vi "HFRR ADV v09.vi"() -> ()   [LabVIEW 2025] (continued)
                # "password"
                # "change password logic"
                n1564 = local read "ENTER CURRENT PASSWORD"() -> (w2733:string)
                n1565 = local read "dipl pwd"() -> (w2727:string)
                n1566 = String To Byte Array(string=w2733) -> (unsigned byte array=w2735:u8[])
                n1567 = String To Byte Array(string=w2727) -> (unsigned byte array=w2728:u8[])
                n1568 = Array Size(array=w2735) -> (size(s)=w2732:i32)
                n1569 = Array Size(array=w2728) -> (size(s)=w2730:i32)
                n1570 = for {
                  N: w2732 -> [_]
                  tunnel: w2735 -> [w2759]
                  tunnel: [w2757] -> w2736 mode=indexing
                  tunnel: w2732 -> [w2751]
                  i -> [w2752]
                  n1571 = Decrement(x=w2751) -> (x-1=w2749:i32)
                  n1572 = Equal?(x=w2752, y=w2749) -> (x = y?=w2750:bool)
                  n1573 = Index Array(array=w2759, index=w2752) -> (element=w2753:u8)
                  n1574 = Number To Decimal String(number=w2753) -> (decimal integer string=w2758:string)  [unwired: 1 in]
                  n1575 = Select(t="", s=w2750, f="\r") -> (s? t:f=w2755:string)
                  n1576 = Concatenate Strings(w2758, w2755) -> (w2757:string)
                }
                n1577 = for {
                  N: w2730 -> [_]
                  tunnel: w2728 -> [w2747]
                  tunnel: [w2745] -> w2729 mode=indexing
                  tunnel: w2730 -> [w2742]
                  i -> [w2743]
                  n1578 = Decrement(x=w2742) -> (x-1=w2741:i32)
                  n1579 = Equal?(x=w2743, y=w2741) -> (x = y?=w2740:bool)
                  n1580 = Index Array(array=w2747, index=w2743) -> (element=w2746:u8)
                  n1581 = Number To Decimal String(number=w2746) -> (decimal integer string=w2744:string)  [unwired: 1 in]
                  n1582 = Select(t="", s=w2740, f="\r") -> (s? t:f=w2737:string)
                  n1583 = Concatenate Strings(w2744, w2737) -> (w2745:string)
                }
                n1584 = local read "string"() -> (w2734:string)
                n1585 = Concatenate Strings(w2729) -> (w2723:string)
                n1586 = Concatenate Strings(w2734) -> (w2731:string)
                n1587 = Concatenate Strings(w2736) -> (w2724:string)
                n1588 = Equal?(x=w2724, y=w2731) -> (x = y?=w2726:bool)
                n1589 = Equal?(x=w2724, y=w2723) -> (x = y?=w2722:bool)
                n1590 = Or(x=w2726, y=w2722) -> (x .or. y?=w2725:bool)
                n1591 = case shown="True" w2725 {
                  frame False {
                  }
                  frame True {
                    n1592 = property on="ENTER THE NEW PASSWORD" class="Str"("Visible"=TRUE) -> ()  [unwired: 2 in, 2 out]
                  }
                }
              }
            }
          }
          frame #2 {
            n1593 = String To Byte Array(string="ENTER THE NEW PASSWORD") -> (unsigned byte array=w2762:u8[])
            n1594 = Search 1D Array(1D array=w2762, element=u8 10) -> (index of element=w2766:i32)  [unwired: 1 in]
            n1595 = Index Array(array=w2762, index=w2766) -> (element=w2764:u8)
            n1596 = Equal?(x=w2764, y=10) -> (x = y?=w2761:bool)
            n1597 = case shown="False" w2761 {
              frame False {
              }
              frame True {
                n1598 = local write "EDIT"(FALSE) -> ()
                n1599 = local write "SrvM CP"(FALSE) -> ()
                n1600 = local read "ENTER THE NEW PASSWORD"() -> (w2769:string)
                n1601 = String To Byte Array(string=w2769) -> (unsigned byte array=w2774:u8[])
                n1602 = Array Size(array=w2774) -> (size(s)=w2771:i32)
                n1603 = for {
                  N: w2771 -> [_]
                  tunnel: w2774 -> [w2787]
                  tunnel: [w2784] -> w2776 mode=indexing
                  tunnel: w2771 -> [w2779]
                  i -> [w2777]
                  n1604 = Decrement(x=w2779) -> (x-1=w2780:i32)
                  n1605 = Equal?(x=w2777, y=w2780) -> (x = y?=w2781:bool)
                  n1606 = Index Array(array=w2787, index=w2777) -> (element=w2786:u8)
                  n1607 = Number To Decimal String(number=w2786) -> (decimal integer string=w2785:string)  [unwired: 1 in]
                  n1608 = Select(t="", s=w2781, f="\r") -> (s? t:f=w2778:string)
                  n1609 = Concatenate Strings(w2785, w2778) -> (w2784:string)
                }
                n1610 = local read "file path"() -> (w2768:path)
                n1611 = Concatenate Strings(w2776) -> (w2770:string)
                n1612 = Delete(path (use dialog)=w2768) -> (deleted path=w2772:path)  [unwired: 4 in, 2 out]
                n1613 = call <vilib>:"Write Characters To File.vi"("append to file? (new file:F)"=FALSE, "character string"=w2770, "file path (dialog if empty)"=w2772) -> ()  [unwired: 2 in, 1 out]
              }
            }
          }
          frame #3 {
            n1614 = case shown="True" "SrvM CP" {
              frame False {
                w2790 = ""
                n1615 = local write "ENTER CURRENT PASSWORD"(w2790) -> ()
                n1616 = local write "ENTER THE NEW PASSWORD"(w2790) -> ()
                n1617 = property on="ENTER CURRENT PASSWORD" class="Str"("Visible"=FALSE) -> ()  [unwired: 2 in, 2 out]
              }
              frame True {
                n1618 = property on="ENTER THE NEW PASSWORD" class="Str"() -> ("Visible"=w2791:bool)  [unwired: 2 in, 2 out]
                n1619 = Not(x=w2791) -> (.not. x?=w2792:bool)
                n1620 = property on="ENTER CURRENT PASSWORD" class="Str"("Visible"=w2792) -> ()  [unwired: 2 in, 2 out]
              }
            }
          }
          frame #4 {
            n1621 = String To Byte Array(string="Password") -> (unsigned byte array=w2799:u8[])
            n1622 = Search 1D Array(1D array=w2799, element=u8 10) -> (index of element=w2797:i32)  [unwired: 1 in]
            n1623 = Index Array(array=w2799, index=w2797) -> (element=w2798:u8)
            n1624 = Equal?(x=w2798, y=10) -> (x = y?=w2794:bool)
            n1625 = case shown="True" w2794 {
              frame False {
              }
              frame True {
                # "password"
                # "password"
                n1626 = local read "Password"() -> (w2812:string)
                n1627 = String To Byte Array(string=w2812) -> (unsigned byte array=w2815:u8[])
                n1628 = String To Byte Array(string="@143$\n") -> (unsigned byte array=w2801:u8[])
                n1629 = Array Size(array=w2815) -> (size(s)=w2810:i32)
                n1630 = Array Size(array=w2801) -> (size(s)=w2806:i32)
                n1631 = for {
                  N: w2810 -> [_]
                  tunnel: w2815 -> [w2849]
                  tunnel: [w2847] -> w2816 mode=indexing
                  tunnel: w2810 -> [w2844]
                  i -> [w2845]
                  n1632 = Decrement(x=w2844) -> (x-1=w2843:i32)
                  n1633 = Index Array(array=w2849, index=w2845) -> (element=w2848:u8)
                  n1634 = Equal?(x=w2845, y=w2843) -> (x = y?=w2842:bool)
                  n1635 = Number To Decimal String(number=w2848) -> (decimal integer string=w2846:string)  [unwired: 1 in]
                  n1636 = Select(t="", s=w2842, f="\r") -> (s? t:f=w2839:string)
                  n1637 = Concatenate Strings(w2846, w2839) -> (w2847:string)
                }
                n1638 = for {
                  N: w2806 -> [_]
                  tunnel: w2801 -> [w2860]
                  tunnel: [w2858] -> w2804 mode=indexing
                  tunnel: w2806 -> [w2855]
                  i -> [w2856]
                  n1639 = Decrement(x=w2855) -> (x-1=w2854:i32)
                  n1640 = Index Array(array=w2860, index=w2856) -> (element=w2859:u8)
                  n1641 = Equal?(x=w2856, y=w2854) -> (x = y?=w2853:bool)
                  n1642 = Number To Decimal String(number=w2859) -> (decimal integer string=w2857:string)  [unwired: 1 in]
                  n1643 = Select(t="", s=w2853, f="\r") -> (s? t:f=w2850:string)
                  n1644 = Concatenate Strings(w2857, w2850) -> (w2858:string)
                }
                n1645 = local read "file path"() -> (w2800:path)
                n1646 = call <vilib>:"Read Characters From File.vi"("file path (dialog if empty)"=w2800) -> ("character string"=w2814:string)  [unwired: 5 in, 3 out]
                "string" <- w2814
                n1647 = flat-sequence {
                  tunnel: [w2817] -> w2811
                  frame #0 {
                    w2817 = ""
                    n1648 = local write "Password"(w2817) -> ()
                  }
                }
                n1649 = Concatenate Strings(w2804) -> (w2805:string)
                n1650 = Concatenate Strings(w2814) -> (w2813:string)
                n1651 = Concatenate Strings(w2816) -> (w2808:string)
                n1652 = Equal?(x=w2808, y=w2813) -> (x = y?=w2803:bool)
                n1653 = Equal?(x=w2808, y=w2805) -> (x = y?=w2809:bool)
                n1654 = Or(x=w2803, y=w2809) -> (x .or. y?=w2802:bool)
                "x = y?" <- w2802
                n1655 = case shown="True" w2802 {
                  selector: w2802 -> [w2819 _]
                  tunnel: w2811 -> [_ _]
                  frame False {
                    n1656 = And(x=w2819, y=TRUE ("Visible")) -> (x .and. y?=w2820:bool)
                    n1657 = property on="message" class="Str"("Visible"=w2820) -> ()  [unwired: 2 in, 2 out]
                  }
                  frame True {
                    n1658 = control-ref of="This VI"() -> (w2831:refnum<vi>)
                    n1659 = property class="VI"(reference=w2831) -> (reference out=w2822:refnum<vi>, error out=w2826:errorcluster, "Panel"=w2830:refnum<vi>)  [unwired: 1 in]
                    n1660 = property on="message" class="Str"("Visible"=FALSE) -> ()  [unwired: 2 in, 2 out]
                    n1661 = property class="Pnl"(reference=w2830, error in=w2826) -> (reference out=w2824:refnum<vi>, error out=w2827:errorcluster, "Panes[]"=w2829:refnum<vi>[])
                    n1662 = for {
                      tunnel: w2829 -> [w2838] mode=indexing
                      tunnel: T17."Always On" ("Horizontal Scrollbar Visibility") -> [w2837]
                      tunnel: w2827 -> [w2834]
                      tunnel: [w2833] -> w2825
                      n1663 = property class="Pane"(reference=w2838, error in=w2834, "HorizScrollbarVisibility"=w2837) -> (reference out=w2835:refnum<vi>, error out=w2836:errorcluster)
                      n1664 = Close Reference(reference=w2835, error in (no error)=w2836) -> (error out=w2833:errorcluster)
                    }
                    n1665 = Close Reference(reference=w2824, error in (no error)=w2825) -> (error out=w2823:errorcluster)
                    n1666 = Close Reference(reference=w2822, error in (no error)=w2823) -> (error out=→"error out 6":errorcluster)
                  }
                }
              }
            }
          }
        }
        n1667 = local read "x = y?"() -> (w2659:bool)
        n1668 = local read "HUMIDITY: 2"() -> (w2661:dbl)
        n1669 = local read "HUMIDITY:"() -> (w2660:dbl)
        n1670 = property on="Port 2 Error" class="Clust (strict)"("Visible"="EDIT") -> ()  [unwired: 2 in, 2 out]
        n1671 = property on="Port 1 Error" class="Clust (strict)"("Visible"="EDIT") -> ()  [unwired: 2 in, 2 out]
        n1672 = case shown="True" "SrvM CP 2" {
          frame False {
          }
          frame True {
            n1673 = local write "SrvM CP 2"(FALSE ("SrvM CP 2")) -> ()
            n1674 = local read "HUMIDITY: 2"() -> (w2700:dbl)
            n1675 = local read "TEMP INTERCEPT: 2"() -> (w2699:dbl)
            n1676 = local read "DISPLACEMENT : 4"() -> (w2703:dbl)
            n1677 = local read "TEMPERATURE : 2"() -> (w2702:dbl)
            n1678 = local read "STROKE GAIN : 2"() -> (w2704:dbl)
            n1679 = local read "FRIC. FORCE : 2"() -> (w2705:dbl)
            n1680 = local read "AIR TEMP INTERCEPT: 2"() -> (w2698:dbl)
            n1681 = local read "AIR TEMPERATURE : 2"() -> (w2701:dbl)
            n1682 = local write "HUMIDITY:"(w2700) -> ()
            n1683 = local write "AIR TEMP INTERCEPT:"(w2699) -> ()
            n1684 = local write "TEMPERATURE :"(w2702) -> ()
            n1685 = local write "FRIC. FORCE :"(w2705) -> ()
            n1686 = local write "STROKE GAIN :"(w2704) -> ()
            n1687 = local write "DISPLACEMENT :"(w2703) -> ()
            n1688 = local write "AIR TEMPERATURE :"(w2701) -> ()
            n1689 = local write "TEMP INTERCEPT:"(w2698) -> ()
          }
        }
        n1690 = case shown="True" "SAVE" {
          frame False {
          }
          frame True {
            n1691 = stacked-sequence {
              seq-local: [w2877 _ _] -> [_ w3041 _]
              frame #0 {
                (unwired) i16 5 ("precision (6)")
                # "[CH1]    - FF\n[CH2]   - TEMPERATURE\n[CH3]    - Humidity\n[CH4]    - AIR TEMP\n[CH5]\\- Visa Uno\n[CH6] \\- Visa Due\n[CH7]  \\- file path\n[CH8]   - Displacement Gain\n[CHA]   - Stroke Gain\n[CHB]   - Stroke PID Gain\n[CHC]   -Language Selection\n[CHD]   -Power +\n[CHE]   -Power_\n[CHF]   -Heater\n[CHG]   -Humidity Wet\n[CHH]   -Humidity Dry\n[CHI]   -Integral Time"
                n1692 = local read "Stroke PID Gains"() -> (w2928:T8)
                n1693 = Unbundle By Name(w2928) -> ("Proportional Gain (Kc)"=w2927:dbl, "Integral Time (Ti, min)"=w2869:dbl)
                n1694 = Number To Fractional String(number=w2869, width (-)=i16 10 ("precision (6)"), precision (6)=i16 5) -> (F-format string=w2873:string)  [unwired: 1 in]
                n1695 = local read "Language Selection"() -> (w2925:enum16{"English", "Russian"})
                n1696 = local read "CH-HUMIDITY WET"() -> (w2883:u16)
                n1697 = local read "CH-HUMIDITY DRY"() -> (w2880:u16)
                n1698 = local read "STROKE GAIN :"() -> (w2861:dbl)
                n1699 = local read "CH-POWER +"() -> (w2892:u16)
                n1700 = local read "CH-POWER -"() -> (w2889:u16)
                n1701 = local read "CH-HEATER"() -> (w2886:u16)
                n1702 = local read "AIR TEMPERATURE :"() -> (w2864:dbl)
                n1703 = Concatenate Strings("[CHI]" ("string"), w2873, "-Integral Time " ("string"), "\r") -> (w2870:string)
                n1704 = local read "DISPLACEMENT :"() -> (w2862:dbl)
                n1705 = local read "TEMPERATURE :"() -> (w2865:dbl)
                n1706 = local read "FRIC. FORCE :"() -> (w2866:dbl)
                n1707 = local read "HUMIDITY:"() -> (w2863:dbl)
                n1708 = Path To String(path="File Path") -> (string=w2950:string)
                n1709 = Number To Fractional String(number=w2861, width (-)=i16 10 ("precision (6)"), precision (6)=i16 5) -> (F-format string=w2941:string)  [unwired: 1 in]
                n1710 = Number To Fractional String(number=w2927, width (-)=i16 10 ("precision (6)"), precision (6)=i16 5) -> (F-format string=w2929:string)  [unwired: 1 in]
                n1711 = Number To Fractional String(number=w2925, width (-)=i16 10 ("precision (6)"), precision (6)=i16 5) -> (F-format string=w2921:string)  [unwired: 1 in]
                n1712 = Number To Fractional String(number=w2892, width (-)=i16 10 ("precision (6)"), precision (6)=i16 5) -> (F-format string=w2915:string)  [unwired: 1 in]
                n1713 = Number To Fractional String(number=w2889, width (-)=i16 10 ("precision (6)"), precision (6)=i16 5) -> (F-format string=w2912:string)  [unwired: 1 in]
                n1714 = Number To Fractional String(number=w2886, width (-)=i16 10 ("precision (6)"), precision (6)=i16 5) -> (F-format string=w2907:string)  [unwired: 1 in]
                n1715 = Number To Fractional String(number=w2883, width (-)=i16 10 ("precision (6)"), precision (6)=i16 5) -> (F-format string=w2904:string)  [unwired: 1 in]
                n1716 = Number To Fractional String(number=w2880, width (-)=i16 10 ("precision (6)"), precision (6)=i16 5) -> (F-format string=w2899:string)  [unwired: 1 in]
                n1717 = local read "Com Port 1"() -> (w2868:refnum<visa-resource-name>)
                n1718 = local read "Com Port 2"() -> (w2867:refnum<visa-resource-name>)
                n1719 = Concatenate Strings(w2950, "\\" ("string")) -> (w2949:string)
                n1720 = Number To Fractional String(number=w2866, width (-)=i16 10 ("precision (6)"), precision (6)=i16 5) -> (F-format string=w2982:string)  [unwired: 1 in]
                n1721 = Number To Fractional String(number=w2865, width (-)=i16 10 ("precision (6)"), precision (6)=i16 5) -> (F-format string=w2981:string)  [unwired: 1 in]
                n1722 = Number To Fractional String(number=w2863, width (-)=i16 10 ("precision (6)"), precision (6)=i16 5) -> (F-format string=w2975:string)  [unwired: 1 in]
                n1723 = Number To Fractional String(number=w2864, width (-)=i16 10 ("precision (6)"), precision (6)=i16 5) -> (F-format string=w2969:string)  [unwired: 1 in]
                n1724 = Number To Fractional String(number=w2862, width (-)=i16 10 ("precision (6)"), precision (6)=i16 5) -> (F-format string=w2942:string)  [unwired: 1 in]
                n1725 = Concatenate Strings("[CHA]" ("string"), w2941, "- Stroke Gain" ("string"), "\r") -> (w2935:string)
                n1726 = Concatenate Strings("[CHB]" ("string"), w2929, "- Stroke PID Gain" ("string"), "\r") -> (w2926:string)
                n1727 = Concatenate Strings("[CHC]" ("string"), w2921, "-Language Selection" ("string"), "\r") -> (w2918:string)
                n1728 = Concatenate Strings("[CHD]" ("string"), w2915, "-Power +" ("string"), "\r") -> (w2897:string)
                n1729 = Concatenate Strings("[CHG]" ("string"), w2904, "-Humidity Wet" ("string"), "\r") -> (w2894:string)
                n1730 = Concatenate Strings("[CHH]" ("string"), w2899, "-Humidity Dry" ("string"), "\r") -> (w2893:string)
                n1731 = Concatenate Strings("[CH1]" ("string"), w2982, " - FF" ("string"), "\r") -> (w2980:string)
                n1732 = Concatenate Strings("[CH2]" ("string"), w2981, " - TEMPERATURE" ("string"), "\r") -> (w2979:string)
                n1733 = Concatenate Strings("[CH3]" ("string"), w2975, " - Humidity" ("string"), "\r") -> (w2972:string)
                n1734 = Concatenate Strings("[CH4]" ("string"), w2969, " - AIR TEMP" ("string"), "\r") -> (w2965:string)
                n1735 = Concatenate Strings("[CH5]" ("string"), w2868, "- Visa Uno" ("string"), "\r") -> (w2958:string)
                n1736 = Concatenate Strings("[CH6]" ("string"), w2867, "- Visa Due" ("string"), "\r") -> (w2953:string)
                n1737 = Concatenate Strings("[CH7]" ("string"), w2949, "- file path" ("string"), "\r") -> (w2952:string)
                n1738 = Concatenate Strings("[CH8]" ("string"), w2942, "- Displacement Gain" ("string"), "\r") -> (w2945:string)
                n1739 = Concatenate Strings("[CHE]" ("string"), w2912, "-Power_" ("string"), "\r") -> (w2896:string)
                n1740 = Concatenate Strings("[CHF]" ("string"), w2907, "-Heater" ("string"), "\r") -> (w2895:string)
                n1741 = Concatenate Strings(w2980, w2979, w2972, w2965, w2958, w2953, w2952, w2945, w2935, w2926, w2918, w2897, w2896, w2895, w2894, w2893, w2870) -> (w2877:string)
                "gain" <- w2877
              }
              frame #1 {
                n1742 = local read "Camera Port :"() -> (w2994:string)
                n1743 = local read "TEMP INTERCEPT:"() -> (w3003:dbl)
                n1744 = local read "Humidity :"() -> (w3002:refnum<visa-resource-name>)
                n1745 = local read "AIR TEMP INTERCEPT:"() -> (w3004:dbl)
                n1746 = local read "LvdtOff"() -> (w3006:dbl)
                n1747 = Number To Fractional String(number=w3003, width (-)=i16 10 ("precision (6)"), precision (6)=i16 5) -> (F-format string=w3029:string)  [unwired: 1 in]
                n1748 = local read "Com Port 3"() -> (w3013:refnum<visa-resource-name>)
                n1749 = Concatenate Strings("[CH8]" ("string"), w2994, "- Visa Camera" ("string"), "\r") -> (w2993:string)
                n1750 = Concatenate Strings("[CH7]" ("string"), w3002, "- Visa Humidity" ("string"), "\r") -> (w2998:string)
                n1751 = Number To Fractional String(number=w3004, width (-)=i16 10 ("precision (6)"), precision (6)=i16 5) -> (F-format string=w3036:string)  [unwired: 1 in]
                n1752 = Number To Fractional String(number=w3006, width (-)=i16 10 ("precision (6)"), precision (6)=i16 5) -> (F-format string=w3010:string)  [unwired: 1 in]
                n1753 = Concatenate Strings("[CHK]" ("string"), w3029, "-TEMP INTERCEPT" ("string"), "\r") -> (w3025:string)
                n1754 = Concatenate Strings("[SNO]" ("string"), "S.NO", "-" ("string"), "\r") -> (w3021:string)
                n1755 = Concatenate Strings("[CHI]" ("string"), w3010, "-LVDT Position Offset" ("string"), "\r") -> (w3005:string)
                n1756 = Concatenate Strings("[CHJ]" ("string"), w3036, "-AIR TEMP INTERCEPT" ("string"), "\r") -> (w3026:string)
                n1757 = Concatenate Strings("[CHL]" ("string"), w3013, "- Visa humid" ("string"), "\r") -> (w3016:string)
                n1758 = String To Path(string="C:\\LAB-IQ\\calibrate WO 2465.dcf") -> (path=w3014:path)
                n1759 = Concatenate Strings(w3041, w3026, w3025, w3021, w3016, w3005, w2998, w2993) -> (w3040:string)
                n1760 = call <vilib>:"Write Characters To File.vi"("append to file? (new file:F)"=FALSE, "character string"=w3040, "file path (dialog if empty)"=w3014) -> ()  [unwired: 2 in, 1 out]
              }
              frame #2 {
                n1761 = local write "Lan flag"(0.0 ("Lan flag")) -> ()
                n1762 = local write "conststatus"(0.0 ("rpm value : 2")) -> ()
                n1763 = local write "SAVE"(FALSE ("OK Button 14")) -> ()
                n1764 = local write "Re-Initialise"(TRUE ("Re-Initialise")) -> ()
              }
            }
          }
        }
        n1765 = And(x="EDIT", y=w2659) -> (x .and. y?=w2657:bool)
        n1766 = local read "DISPLACEMENT : 4"() -> (w2670:dbl)
        n1767 = local read "TEMPERATURE : 2"() -> (w2668:dbl)
        n1768 = local read "STROKE GAIN : 2"() -> (w2674:dbl)
        n1769 = local read "DISPLACEMENT :"() -> (w2669:dbl)
        n1770 = local read "FRIC. FORCE : 2"() -> (w2677:dbl)
        n1771 = local read "TEMPERATURE :"() -> (w2666:dbl)
        n1772 = local read "STROKE GAIN :"() -> (w2673:dbl)
        n1773 = local read "FRIC. FORCE :"() -> (w2676:dbl)
        n1774 = case shown="True" w2657 {
          tunnel: [u8 2 ("Disabled") u8 0 ("Disabled")] -> w2656
          tunnel: [w3046 TRUE ("Visible")] -> w2655
          frame False {
            w3046 = FALSE ("Visible")
            n1775 = local write "EDIT 2"(w3046) -> ()
          }
          frame True {
          }
        }
        n1776 = Subtract(x=w2661, y=w2660) -> (x-y=w2662:dbl)
        n1777 = local read "AIR TEMPERATURE : 2"() -> (w2665:dbl)
        n1778 = local read "AIR TEMPERATURE :"() -> (w2664:dbl)
        n1779 = Divide(x=w2662, y=w2660) -> (x/y=w2684:dbl)
        n1780 = Subtract(x=w2677, y=w2676) -> (x-y=w2675:dbl)
        n1781 = Subtract(x=w2668, y=w2666) -> (x-y=w2667:dbl)
        n1782 = Subtract(x=w2674, y=w2673) -> (x-y=w2672:dbl)
        n1783 = Subtract(x=w2670, y=w2669) -> (x-y=w2671:dbl)
        n1784 = Subtract(x=w2665, y=w2664) -> (x-y=w2663:dbl)
        n1785 = Divide(x=w2675, y=w2676) -> (x/y=w2695:dbl)
        n1786 = Divide(x=w2667, y=w2666) -> (x/y=w2688:dbl)
        n1787 = Divide(x=w2672, y=w2673) -> (x/y=w2692:dbl)
        n1788 = Divide(x=w2671, y=w2669) -> (x/y=w2691:dbl)
        n1789 = Multiply(x=w2684, y=100.0) -> (x*y=→"HUMIDITY  Calibration Error":dbl)
        n1790 = Divide(x=w2663, y=w2664) -> (x/y=w2687:dbl)
        n1791 = Multiply(x=w2695, y=100.0) -> (x*y=→"FRIC. FORCE Calibration Error":dbl)
        n1792 = Multiply(x=w2688, y=100.0) -> (x*y=→"TEMPERATURE  Calibration Error":dbl)
        n1793 = Multiply(x=w2692, y=100.0) -> (x*y=→"STROKE Calibration Error":dbl)
        n1794 = Multiply(x=w2691, y=100.0) -> (x*y=→"DISPLACEMENT  Calibration Error":dbl)
        n1795 = property on="EDIT 2" class="Bool (strict)"("Visible"=w2655) -> ()  [unwired: 2 in, 2 out]
        n1796 = property on="SAVE" class="Bool (strict)"("Visible"=w2655) -> ()  [unwired: 2 in, 2 out]
        n1797 = property on="SrvM CP" class="Bool (strict)"("Disabled"=w2656) -> ()  [unwired: 2 in, 2 out]
        n1798 = property on="visa due" class="CmbBox"("Disabled"=w2656) -> ()  [unwired: 2 in, 2 out]
        n1799 = property on="LvdtOff" class="DigNum (strict)"("Disabled"=w2656) -> ()  [unwired: 2 in, 2 out]
        n1800 = property on="File Path" class="Path"("Disabled"=w2656) -> ()  [unwired: 2 in, 2 out]
        n1801 = Multiply(x=w2687, y=100.0) -> (x*y=→"AIR TEMPERATURE  Calibration Error":dbl)
        n1802 = property on="Tab Control" class="TabCtl (strict)"("Visible"=w2655) -> ()  [unwired: 2 in, 2 out]
        n1803 = property on="Language Selection" class="Enum (strict)"("Visible"=w2655) -> ()  [unwired: 2 in, 2 out]
        n1804 = property on="Tab Control 7" class="TabCtl (strict)"("Disabled"=w2656) -> ()  [unwired: 2 in, 2 out]
        n1805 = property on="AIR TEMP INTERCEPT:" class="DigNum (strict)"("Disabled"=w2656) -> ()  [unwired: 2 in, 2 out]
        n1806 = property on="CH-POWER -" class="DigNum (strict)"("Disabled"=w2656) -> ()  [unwired: 2 in, 2 out]
        n1807 = property on="CH-POWER +" class="DigNum (strict)"("Disabled"=w2656) -> ()  [unwired: 2 in, 2 out]
        n1808 = property on="AIR TEMPERATURE :" class="DigNum (strict)"("Disabled"=w2656) -> ()  [unwired: 2 in, 2 out]
        n1809 = property on="STROKE GAIN :" class="DigNum (strict)"("Disabled"=w2656) -> ()  [unwired: 2 in, 2 out]
        n1810 = property on="SPEED OUT:" class="DigNum (strict)"("Disabled"=w2656) -> ()  [unwired: 2 in, 2 out]
        n1811 = property on="CH-HUMIDITY DRY" class="DigNum (strict)"("Disabled"=w2656) -> ()  [unwired: 2 in, 2 out]
        n1812 = property on="HUMIDITY:" class="DigNum (strict)"("Disabled"=w2656) -> ()  [unwired: 2 in, 2 out]
        n1813 = property on="CH-HUMIDITY WET" class="DigNum (strict)"("Disabled"=w2656) -> ()  [unwired: 2 in, 2 out]
        n1814 = property on="Stroke PID Gains" class="Clust (strict)"("Disabled"=w2656) -> ()  [unwired: 2 in, 2 out]
        n1815 = property on="TEMPERATURE :" class="DigNum (strict)"("Disabled"=w2656) -> ()  [unwired: 2 in, 2 out]
        n1816 = property on="DISPLACEMENT :" class="DigNum (strict)"("Disabled"=w2656) -> ()  [unwired: 2 in, 2 out]
        n1817 = property on="CH-HEATER" class="DigNum (strict)"("Disabled"=w2656) -> ()  [unwired: 2 in, 2 out]
        n1818 = property on="TEMP INTERCEPT:" class="DigNum (strict)"("Disabled"=w2656) -> ()  [unwired: 2 in, 2 out]
        n1819 = property on="FRIC. FORCE :" class="DigNum (strict)"("Disabled"=w2656) -> ()  [unwired: 2 in, 2 out]
      }
    }
    n1820 = local read "RUN"() -> (w2051:bool)
    n1821 = local read "RUN"() -> (w2049:bool)
    n1822 = disable-structure shown="Disabled" {
      disable-tunnel: [w2066 _] -> w2031
      disable-tunnel: [w2065 _] -> w2029
      frame Disabled {
        n1823 = local read "Temperature before test"() -> (w2059:dbl)
        n1824 = local read "Temperature after test"() -> (w2072:dbl)
        n1825 = case shown="True" "Save Results" {
          frame False {
          }
          frame True {
            w2088 = "\r"
            n1826 = local write "Save Results"(FALSE ("OK Button 5")) -> ()
            n1827 = local read "Temperature before test"() -> (w2126:dbl)
            n1828 = local read "Temperature after test"() -> (w2128:dbl)
            n1829 = local read "Humidity before test"() -> (w2125:dbl)
            n1830 = local read "Humidity after test"() -> (w2127:dbl)
            n1831 = local read "WS1.4"() -> (w2132:dbl)
            n1832 = local read "AVP"() -> (w2130:dbl)
            n1833 = Number To Fractional String(number=w2132, width (-)=i16 6, precision (6)=i16 1) -> (F-format string=w2092:string)  [unwired: 1 in]
            n1834 = local read "MWSD"() -> (w2129:dbl)
            n1835 = local read "String"() -> (w2121:string)
            n1836 = local read "FILE"() -> (w2124:string)
            n1837 = local read "HCF"() -> (w2131:dbl)
            n1838 = Number To Fractional String(number=w2125, width (-)=i16 6, precision (6)=i16 1) -> (F-format string=w2117:string)  [unwired: 1 in]
            n1839 = Number To Fractional String(number=w2126, width (-)=i16 6, precision (6)=i16 1) -> (F-format string=w2114:string)  [unwired: 1 in]
            n1840 = Number To Fractional String(number=w2127, width (-)=i16 6, precision (6)=i16 1) -> (F-format string=w2110:string)  [unwired: 1 in]
            n1841 = Number To Fractional String(number=w2128, width (-)=i16 6, precision (6)=i16 1) -> (F-format string=w2106:string)  [unwired: 1 in]
            n1842 = Number To Fractional String(number=w2130, width (-)=i16 6, precision (6)=i16 3) -> (F-format string=w2099:string)  [unwired: 1 in]
            n1843 = Concatenate Strings(w2121, w2124) -> (w2143:string)
            n1844 = Number To Fractional String(number=w2129, width (-)=i16 6, precision (6)=i16 1) -> (F-format string=w2103:string)  [unwired: 1 in]
            n1845 = Number To Fractional String(number=w2131, width (-)=i16 6, precision (6)=i16 2) -> (F-format string=w2097:string)  [unwired: 1 in]
            n1846 = Concatenate Strings("(" ("string"), w2092, ")Microns" ("string")) -> (w2091:string)
            n1847 = local read "REMARKS"() -> (w2123:string)
            "REMARKS 2" <- w2123
            n1848 = Concatenate Strings("(" ("string"), w2117, " ) % RH," ("string")) -> (w2118:string)
            n1849 = Concatenate Strings(w2097, ")" ("string")) -> (w2095:string)
            n1850 = Concatenate Strings("(" ("string"), w2114, ")  Deg C ," ("string")) -> (w2113:string)
            n1851 = Concatenate Strings("(" ("string"), w2110, " ) % RH," ("string")) -> (w2109:string)
            n1852 = Concatenate Strings("(" ("string"), w2106, ")  Deg C ," ("string")) -> (w2105:string)
            n1853 = Concatenate Strings("(" ("string"), w2103, ")  Microns," ("string")) -> (w2102:string)
            n1854 = Concatenate Strings("(" ("string"), w2099, ")  kPa," ("string")) -> (w2089:string)
            n1855 = Concatenate Strings(w2143, ".dwm" ("Substring")) -> (w2141:string)
            n1856 = String To Path(string=w2141) -> (path=w2140:path)
            n1857 = Concatenate Strings(w2123, w2088, " Humidity before test= " ("Substring"), w2118, w2088, " Temperature before test = " ("Substring"), w2113, w2088, " Humidity after test= " ("Substring"), w2109, w2088, "Temperature after test = " ("Substring"), w2105, w2088, "MSD = " ("Substring"), w2102, w2088, "  AVP = " ("Substring"), w2089, w2088, "  HCF                     =( " ("Substring"), w2095, w2088, " WS1.4                  = " ("Substring"), w2091, w2088) -> (w2087:string)
            "data" <- w2087
            n1858 = call <vilib>:"Write Characters To File.vi"("append to file? (new file:F)"=FALSE, "character string"=w2087, "file path (dialog if empty)"=w2140) -> ()  [unwired: 2 in, 1 out]
            n1859 = Match Pattern(string=w2087, regular expression="!") -> (after substring=→"export":string)  [unwired: 1 in, 3 out]
          }
        }
        n1860 = Add(x=231.864, y=w2059) -> (x+y=w2056:dbl)
        n1861 = Add(x=231.864, y=w2072) -> (x+y=w2069:dbl)
        n1862 = Divide(x=1705.984, y=w2056) -> (x/y=w2057:dbl)
        n1863 = Divide(x=1705.984, y=w2069) -> (x/y=w2070:dbl)
        n1864 = local read "Humidity before test"() -> (w2061:dbl)
        n1865 = local read "Humidity after test"() -> (w2074:dbl)
        n1866 = Subtract(x=8.017352 ("y"), y=w2057) -> (x-y=w2083:dbl)
        n1867 = Subtract(x=8.017352 ("y"), y=w2070) -> (x-y=w2077:dbl)
        n1868 = expression code="10**y"(w2083) -> (w2063:dbl)
        n1869 = expression code="10**y"(w2077) -> (w2076:dbl)
        n1870 = Multiply(x=w2061, y=w2063) -> (x*y=w2062:dbl)
        n1871 = Multiply(x=w2074, y=w2076) -> (x*y=w2075:dbl)
        n1872 = Divide(x=w2062, y=750.0) -> (x/y=w2078:dbl)
        n1873 = Divide(x=w2075, y=750.0) -> (x/y=w2079:dbl)
        n1874 = Add(x=w2078, y=w2079) -> (x+y=w2080:dbl)
        n1875 = Divide(x=w2080, y=2.0) -> (x/y=w2082:dbl)
        n1876 = local write "AVP"(w2082) -> ()
        n1877 = Subtract(x=1.4, y=w2082) -> (x-y=w2065:dbl)
        n1878 = local read "HCF"() -> (w2066:dbl)
      }
      frame Enabled {
      }
    }
    n1879 = case shown="True" "EDIT 3" {
      frame False {
      }
      frame True {
        n1880 = local write "EDIT 3"(FALSE ("EDIT 3")) -> ()
        n1881 = local write "Main Tab"(T2."About" ("Main Tab")) -> ()
      }
    }
    n1882 = case shown="True" w2037 {
      frame False {
      }
      frame True {
        n1883 = local write "Re-Initialise"(FALSE ("Re-Initialise")) -> ()
      }
    }
    n1884 = case shown="False" w2051 {
      frame False {
        n1885 = local read "stopT"() -> (w3053:bool)
        n1886 = case shown="True" w3053 {
          frame False {
          }
          frame True {
            w3054 = FALSE
            n1887 = local write "stopT"(w3054) -> ()
            n1888 = local write "st enable"(w3054) -> ()
          }
        }
      }
      frame True {
        "stopT" <- TRUE
      }
    }
    n1889 = case shown="True" w2049 {
      frame False {
      }
      frame True {
      }
    }
    n1890 = case shown="True" w2039 {
      frame False {
        n1891 = property on="Password 2" class="Str"("Visible"=FALSE) -> ()  [unwired: 2 in, 2 out]
        n1892 = local write "Password 2"("" ("Password")) -> ()
      }
      frame True {
        n1893 = property on="Password 2" class="Str"("Visible"=TRUE) -> ()  [unwired: 2 in, 2 out]
        n1894 = Equal?(x="Password 2", y="HFRR1234") -> (x = y?=w2172:bool)
        n1895 = case shown="True" w2172 {
          tunnel: "Password 2" -> [w2175 _]
          frame False {
            n1896 = String Length(string=w2175) -> (length=w2176:i32)
            n1897 = Greater Than 0?(x=w2176) -> (x > 0?=w2174:bool)
            n1898 = case shown="False" w2174 {
              frame False {
                n1899 = property on="Password 2" class="Str"("Caption.Text"="Password (Advance Setting)") -> ()  [unwired: 2 in, 2 out]
              }
              frame True {
                n1900 = property on="Password 2" class="Str"("Caption.Text"="Incorrect Password!") -> ()  [unwired: 2 in, 2 out]
              }
            }
          }
          frame True {
            n1901 = local write "EDIT 2"(FALSE ("EDIT 2")) -> ()
            n1902 = local write "Password 2"("" ("Password")) -> ()
            n1903 = local write "Main Tab"(T2."Advance" ("Main Tab")) -> ()
            n1904 = local write "Main Dashboard Buttons"(T1."Advance" ("Main Dashboard Buttons")) -> ()
          }
        }
      }
    }
    n1905 = case shown="True" "Prog Uno" {
      frame False {
      }
      frame True {
        n1906 = stacked-sequence {
          frame #0 {
            n1907 = Delete(path (use dialog)=path "C:/LAB-IQ-NXT/UNOCOMPILE.bat" ("working directory")) -> ()  [unwired: 4 in, 3 out]
          }
          frame #1 {
            n1908 = local read "Com Port 1"() -> (w2637:refnum<visa-resource-name>)
            n1909 = Concatenate Strings("cmd.exe /c \"mode " ("command line"), w2637, ":1200,n,8,1\"\n" ("command line")) -> (w2642:string)
            n1910 = Concatenate Strings(w2642, "CD\\\nCD WinDucom\navrdude -C avrdude.conf -v -patmega328p -carduino -P" ("command line"), w2637, " -b115200 -D -Uflash:w:UNO_V20.hex:i\n" ("command line"), "\r") -> (w2644:string)
            "STR" <- w2644
            n1911 = call <vilib>:"Write Characters To File.vi"("append to file? (new file:F)"=FALSE, "character string"=w2644, "file path (dialog if empty)"=path "C:/LAB-IQ/UNOCOMPILE.bat" ("working directory")) -> ()  [unwired: 2 in, 1 out]
          }
          frame #2 {
            n1912 = disable-structure shown="Disabled" {
              frame Disabled {
                w2648 = "cmd.exe  /c \"C:\\LAB-IQ-NXT\\UNOCOMPILE.bat\"" ("string")
                n1913 = local write "Prog Uno"(FALSE ("run minimized? (F)")) -> ()
                n1914 = call <vilib>:"System Exec.vi"("expected output size  (4096)"=u32 65535, "run minimized? (F)"=FALSE, "wait until completion? (T)"=TRUE ("run minimized? (F)"), "working directory"=path "C:/LAB-IQ-NXT", "standard input"=w2648, "command line"=w2648) -> ("error out"=w2647:errorcluster, "standard output"=→"String 42":string)  [unwired: 2 in, 2 out]
                "error out 3" <- w2647
                n1915 = flat-sequence {
                  tunnel: w2647 -> [_]
                  frame #0 {
                  }
                }
              }
              frame Enabled {
              }
            }
          }
        }
      }
    }
    n1916 = case shown="\"ASTM D6079\", Default" "TEST STANDARD" {
      tunnel: [2.0 ("Set Temp") 0.0 ("Set Temp") 2.0 ("Set Temp") 0.0 ("Set Temp")] -> w2040
      frame "ASTM D6079", Default {
        w2594 = 50.0 ("Hz")
        w2595 = 53.0 ("Set Rh")
        w2597 = 1.0 ("Set Strk")
        w2596 = 60.0 ("Set Temp")
        # "astm hide"
        n1917 = local write "NORMAL LOAD"(2.0 ("NORMAL LOAD")) -> ()
        n1918 = local write "Set Strk"(w2597) -> ()
        n1919 = local write "Set Hz"(w2594) -> ()
        n1920 = local write "Set Temp"(w2596) -> ()
        n1921 = local write "Set Rh"(w2595) -> ()
        n1922 = local write "test time"(75.0 ("test time")) -> ()
        n1923 = local write "Set Stroke:"(w2597) -> ()
        n1924 = local write "Set Humidity:"(w2595) -> ()
        n1925 = local write "Set Frequency:"(w2594) -> ()
        n1926 = local write "Set Temperature:"(w2596) -> ()
        "Test Standard" <- "ASTM D6079" ("Test Standard 2")
      }
      frame "ISO 12156" {
        n1927 = local write "Set Strk"(1.0 ("Set Strk")) -> ()
        n1928 = local write "NORMAL LOAD"(2.0 ("NORMAL LOAD")) -> ()
        n1929 = local write "Set Temp"(60.0 ("Set Temp")) -> ()
        n1930 = local write "test time"(75.0 ("test time")) -> ()
        n1931 = local write "Set Hz"(50.0 ("Hz")) -> ()
        n1932 = local write "Set Rh"(53.0 ("Set Rh")) -> ()
      }
      frame "CEC F-096-A-06" {
        n1933 = local write "Set Strk"(1.0 ("Set Strk")) -> ()
        n1934 = local write "NORMAL LOAD"(2.0 ("NORMAL LOAD")) -> ()
        n1935 = local write "Set Temp"(60.0 ("Set Temp")) -> ()
        n1936 = local write "test time"(75.0 ("test time")) -> ()
        n1937 = local write "Set Hz"(50.0 ("Hz")) -> ()
        n1938 = local write "Set Rh"(53.0 ("Set Rh")) -> ()
      }
      frame "Custom" {
      }
    }
    n1939 = case shown="True" "Prog Due" {
      frame False {
      }
      frame True {
        n1940 = stacked-sequence {
          frame #0 {
            n1941 = Delete(path (use dialog)=path "C:/LAB-IQ/DUECOMPILE.bat" ("working directory")) -> ()  [unwired: 4 in, 3 out]
          }
          frame #1 {
            n1942 = disable-structure shown="Disabled" {
              frame Disabled {
                n1943 = local read "visa due"() -> (w2619:string)
                n1944 = Concatenate Strings("cmd.exe /c \"mode " ("command line"), w2619, ":1200,n,8,1\"\n" ("command line")) -> (w2624:string)
                n1945 = Concatenate Strings(w2624, "CD\\\nCD WinDucom\nTIMEOUT 1\n bossac.exe -i -d --port=" ("command line"), w2619, " -U false -e -w -v -b DUE.bin -R\n" ("command line"), "\r") -> (w2626:string)
                "concatenated string 2" <- w2626
                n1946 = call <vilib>:"Write Characters To File.vi"("append to file? (new file:F)"=FALSE, "character string"=w2626, "file path (dialog if empty)"=path "C:/LAB-IQ-NXT/DUECOMPILE.bat" ("working directory")) -> ()  [unwired: 2 in, 1 out]
              }
              frame Enabled {
              }
            }
          }
          frame #2 {
            # "C:\\LAB-IQ-NXT\\DUECOMPILE.bat"
            n1947 = disable-structure shown="Disabled" {
              frame Disabled {
                w2631 = "cmd.exe  /c \"C:\\LAB-IQ-NXT\\DUECOMPILE.bat\"" ("string")
                n1948 = call <vilib>:"System Exec.vi"("expected output size  (4096)"=u32 65535, "run minimized? (F)"=FALSE, "wait until completion? (T)"=TRUE ("run minimized? (F)"), "working directory"=path "C:/LAB-IQ-NXT", "standard input"=w2631, "command line"=w2631) -> ("error out"=w2630:errorcluster, "standard output"=→"String 44":string)  [unwired: 2 in, 2 out]
                "error out 4" <- w2630
                n1949 = flat-sequence {
                  tunnel: w2630 -> [_]
                  frame #0 {
                  }
                }
              }
              frame Enabled {
              }
            }
            n1950 = local write "Prog Due"(FALSE ("Prog Due")) -> ()
          }
        }
      }
    }
    n1951 = Or(x=w2036, y=w2034) -> (x .or. y?=w2035:bool)
    n1952 = case shown="\"About\"" w2033 {
      tunnel: [T22."Acquire" ("Main Tab") T22."Compare Files" ("Main Tab") T22."About" ("Main Tab")] -> w2047
      frame "Acquire", Default {
      }
      frame "Compare Files" {
      }
      frame "About" {
      }
    }
    n1953 = Or(x=w2041, y="OPEN") -> (x .or. y?=w2042:bool)
    n1954 = case shown="True" w2042 {
      tunnel: w2041 -> [_ w2183]
      frame False {
      }
      frame True {
        n1955 = stacked-sequence {
          tunnel: w2183 -> [_ w2250 _ _]
          frame #0 {
            w2199 = "  " ("String 6")
            n1956 = local write "OPEN"(FALSE ("open")) -> ()
            n1957 = local read "string1 2"() -> (w2187:string)
            n1958 = local read "string1 3"() -> (w2186:string)
            n1959 = local read "string1 4"() -> (w2185:string)
            n1960 = property on="OPEN" class="Bool (strict)"("Visible"=FALSE) -> ()  [unwired: 2 in, 2 out]
            n1961 = local write "String 6"(w2199) -> ()
            n1962 = local write "String 7"(w2199) -> ()
            n1963 = local write "String 8"(w2199) -> ()
            n1964 = local write "String 12"(w2199) -> ()
            n1965 = local read "OK Button 16"() -> (w2184:bool)
            n1966 = String To Path(string=w2187) -> (path=w2195:path)
            n1967 = String To Path(string=w2186) -> (path=w2194:path)
            n1968 = String To Path(string=w2185) -> (path=w2193:path)
            n1969 = case shown="True" w2184 {
              tunnel: [w2200 w2201] -> w2188
              frame False {
                n1970 = local read "string1"() -> (w2200:string)
              }
              frame True {
                n1971 = local read "String Indicator 4"() -> (w2201:string)
              }
            }
            n1972 = Open/Create/Replace File "Open File"(file path (use dialog)=w2195) -> (refnum out=w2191:refnum<file>)  [unwired: 5 in, 2 out]
            n1973 = Open/Create/Replace File "Open File"(file path (use dialog)=w2194) -> (refnum out=w2190:refnum<file>)  [unwired: 5 in, 2 out]
            n1974 = Open/Create/Replace File "Open File"(file path (use dialog)=w2193) -> (refnum out=w2189:refnum<file>)  [unwired: 5 in, 2 out]
            n1975 = while {
              tunnel: w2191 -> [w2213]
              i -> [w2209]
              stop <- w2208 continue-if-true
              (unwired) TRUE ("line mode (F)")
              n1976 = Read from Text File "Read File"(file (use dialog)=w2213) -> (text=w2210:string)  [unwired: 3 in, 3 out]
              n1977 = local write "Numeric 11"(w2209) -> ()
              n1978 = String Length(string=w2210) -> (length=w2212:i32)
              n1979 = Greater?(x=w2212, y=1) -> (0:w2208:bool)
            }
            n1980 = while {
              tunnel: w2190 -> [w2219]
              i -> [w2215]
              stop <- w2214 continue-if-true
              (unwired) TRUE ("line mode (F)")
              n1981 = Read from Text File "Read File"(file (use dialog)=w2219) -> (text=w2216:string)  [unwired: 3 in, 3 out]
              n1982 = local write "Numeric 12"(w2215) -> ()
              n1983 = String Length(string=w2216) -> (length=w2218:i32)
              n1984 = Greater?(x=w2218, y=1) -> (0:w2214:bool)
            }
            n1985 = while {
              tunnel: w2189 -> [w2225]
              i -> [w2221]
              stop <- w2220 continue-if-true
              (unwired) TRUE ("line mode (F)")
              n1986 = Read from Text File "Read File"(file (use dialog)=w2225) -> (text=w2222:string)  [unwired: 3 in, 3 out]
              n1987 = local write "Numeric 13"(w2221) -> ()
              n1988 = String Length(string=w2222) -> (length=w2224:i32)
              n1989 = Greater?(x=w2224, y=1) -> (0:w2220:bool)
            }
            n1990 = String To Path(string=w2188) -> (path=w2196:path)
            n1991 = Open/Create/Replace File "Open File"(file path (use dialog)=w2196) -> (refnum out=w2192:refnum<file>)  [unwired: 5 in, 2 out]
            n1992 = while {
              tunnel: w2192 -> [w2207]
              i -> [w2203]
              stop <- w2202 continue-if-true
              (unwired) TRUE ("line mode (F)")
              n1993 = Read from Text File "Read File"(file (use dialog)=w2207) -> (text=w2204:string)  [unwired: 3 in, 3 out]
              n1994 = local write "Numeric 8"(w2203) -> ()
              n1995 = String Length(string=w2204) -> (length=w2206:i32)
              n1996 = Greater?(x=w2206, y=1) -> (0:w2202:bool)
            }
          }
          frame #1 {
            w2377 = FALSE ("ACTUAL   MERGE")
            # "Sample Temp"
            # "ECR"
            # "COF"
            # "Time\nCOF\nFF\nTemp"
            n1997 = case shown="True" w2250 {
              tunnel: [w2397 w2398] -> w2251
              frame False {
                n1998 = local read "string1"() -> (w2397:string)
              }
              frame True {
                n1999 = local read "String Indicator 4"() -> (w2398:string)
              }
            }
            n2000 = local read "string1 3"() -> (w2295:string)
            n2001 = String To Path(string=w2251) -> (path=w2382:path)
            n2002 = String To Path(string=w2295) -> (path=w2393:path)
            n2003 = local read "Numeric 12"() -> (w2379:i32)
            n2004 = local read "Numeric 8"() -> (w2381:i32)
            n2005 = local read "string1 2"() -> (w2296:string)
            n2006 = local read "string1 4"() -> (w2294:string)
            n2007 = Open/Create/Replace File "Open File"(file path (use dialog)=w2382) -> (refnum out=w2396:refnum<file>, error out=w2395:errorcluster)  [unwired: 5 in, 1 out]
            n2008 = Open/Create/Replace File "Open File"(file path (use dialog)=w2393) -> (refnum out=w2389:refnum<file>, error out=w2390:errorcluster)  [unwired: 5 in, 1 out]
            n2009 = for {
              N: w2381 -> [_]
              tunnel: w2396 -> [w2544]
              tunnel: w2395 -> [w2543]
              tunnel: [w2533] -> w2308 mode=indexing
              tunnel: [w2531] -> w2365 mode=indexing
              tunnel: [w2532] -> w2360 mode=indexing
              tunnel: w2377 -> [_]
              tunnel: [w2525] -> w2362 mode=indexing
              tunnel: [w2521] -> w2331 mode=indexing
              tunnel: [w2517] -> w2306 mode=indexing
              tunnel: [w2513] -> w2287 mode=indexing
              tunnel: [w2508] -> w2247 mode=indexing
              (unwired) TRUE ("line mode (F)")
              # "freq"
              # "Stroke"
              # "Time"
              # "CoF"
              # "Humidity"
              # "Temp"
              # "Air Temp"
              # "ECR"
              n2010 = Read from Text File "Read File"(file (use dialog)=w2544, error in=w2543) -> (text=w2509:string)  [unwired: 2 in, 3 out]
              n2011 = local write "String 6"(w2509) -> ()
              n2012 = String Subset(string=w2509, offset (0)=0, length (rest)=14 ("length (rest)")) -> (substring=w2537:string)
              n2013 = String Subset(string=w2509, offset (0)=35, length (rest)=9 ("length (rest)")) -> (substring=w2534:string)
              n2014 = String Subset(string=w2509, offset (0)=15, length (rest)=9 ("length (rest)")) -> (substring=w2540:string)
              n2015 = Fract/Exp String To Number(string=w2537) -> (number=w2533:dbl)  [unwired: 3 in, 1 out]
              n2016 = Fract/Exp String To Number(string=w2534) -> (number=w2532:dbl)  [unwired: 3 in, 1 out]
              n2017 = Fract/Exp String To Number(string=w2540) -> (number=w2531:dbl)  [unwired: 3 in, 1 out]
              n2018 = String Subset(string=w2509, offset (0)=85, length (rest)=9 ("length (rest)")) -> (substring=w2510:string)
              n2019 = String Subset(string=w2509, offset (0)=25, length (rest)=9 ("length (rest)")) -> (substring=w2516:string)
              n2020 = String Subset(string=w2509, offset (0)=55, length (rest)=9 ("length (rest)")) -> (substring=w2518:string)
              n2021 = String Subset(string=w2509, offset (0)=45, length (rest)=9 ("length (rest)")) -> (substring=w2524:string)
              n2022 = String Subset(string=w2509, offset (0)=65, length (rest)=9 ("length (rest)")) -> (substring=w2530:string)
              n2023 = Fract/Exp String To Number(string=w2516) -> (number=w2513:dbl)  [unwired: 3 in, 1 out]
              n2024 = Fract/Exp String To Number(string=w2510) -> (number=w2508:dbl)  [unwired: 3 in, 1 out]
              n2025 = Fract/Exp String To Number(string=w2518) -> (number=w2517:dbl)  [unwired: 3 in, 1 out]
              n2026 = Fract/Exp String To Number(string=w2524) -> (number=w2521:dbl)  [unwired: 3 in, 1 out]
              n2027 = Fract/Exp String To Number(string=w2530) -> (number=w2527:dbl)  [unwired: 3 in, 1 out]
              n2028 = Add(x=w2527, y=0.0) -> (x+y=w2525:dbl)
            }
            n2029 = for {
              N: w2379 -> [_]
              tunnel: w2390 -> [w2470]
              tunnel: w2389 -> [w2469]
              tunnel: [w2459] -> w2348 mode=indexing
              tunnel: [w2457] -> w2346 mode=indexing
              tunnel: [w2458] -> w2342 mode=indexing
              tunnel: w2377 -> [_]
              tunnel: [w2451] -> w2344 mode=indexing
              tunnel: [w2447] -> w2326 mode=indexing
              tunnel: [w2443] -> w2302 mode=indexing
              tunnel: [w2440] -> w2283 mode=indexing
              tunnel: [w2436] -> w2242 mode=indexing
              (unwired) 9 ("length (rest)")
              (unwired) 9 ("length (rest)")
              (unwired) TRUE ("line mode (F)")
              n2030 = Read from Text File "Read File"(file (use dialog)=w2469, error in=w2470) -> (text=w2437:string)  [unwired: 2 in, 3 out]
              n2031 = local write "String 8"(w2437) -> ()
              n2032 = String Subset(string=w2437, offset (0)=85) -> (substring=w2439:string)  [unwired: 1 in]
              n2033 = String Subset(string=w2437, offset (0)=35, length (rest)=9 ("length (rest)")) -> (substring=w2460:string)
              n2034 = String Subset(string=w2437, offset (0)=55, length (rest)=9 ("length (rest)")) -> (substring=w2445:string)
              n2035 = String Subset(string=w2437, offset (0)=25) -> (substring=w2441:string)  [unwired: 1 in]
              n2036 = String Subset(string=w2437, offset (0)=15, length (rest)=9 ("length (rest)")) -> (substring=w2466:string)
              n2037 = String Subset(string=w2437, offset (0)=0, length (rest)=14 ("length (rest)")) -> (substring=w2463:string)
              n2038 = String Subset(string=w2437, offset (0)=45, length (rest)=9 ("length (rest)")) -> (substring=w2450:string)
              n2039 = String Subset(string=w2437, offset (0)=65, length (rest)=9 ("length (rest)")) -> (substring=w2456:string)
              n2040 = Fract/Exp String To Number(string=w2439) -> (number=w2436:dbl)  [unwired: 3 in, 1 out]
              n2041 = Fract/Exp String To Number(string=w2460) -> (number=w2458:dbl)  [unwired: 3 in, 1 out]
              n2042 = Fract/Exp String To Number(string=w2445) -> (number=w2443:dbl)  [unwired: 3 in, 1 out]
              n2043 = Fract/Exp String To Number(string=w2441) -> (number=w2440:dbl)  [unwired: 3 in, 1 out]
              n2044 = Fract/Exp String To Number(string=w2466) -> (number=w2457:dbl)  [unwired: 3 in, 1 out]
              n2045 = Fract/Exp String To Number(string=w2463) -> (number=w2459:dbl)  [unwired: 3 in, 1 out]
              n2046 = Fract/Exp String To Number(string=w2450) -> (number=w2447:dbl)  [unwired: 3 in, 1 out]
              n2047 = Fract/Exp String To Number(string=w2456) -> (number=w2453:dbl)  [unwired: 3 in, 1 out]
              n2048 = Add(x=w2453, y=0.0) -> (x+y=w2451:dbl)
            }
            n2049 = String To Path(string=w2296) -> (path=w2394:path)
            n2050 = String To Path(string=w2294) -> (path=w2388:path)
            n2051 = local read "Numeric 11"() -> (w2378:i32)
            n2052 = local read "Numeric 13"() -> (w2380:i32)
            n2053 = Open/Create/Replace File "Open File"(file path (use dialog)=w2394) -> (refnum out=w2392:refnum<file>, error out=w2391:errorcluster)  [unwired: 5 in, 1 out]
            n2054 = Open/Create/Replace File "Open File"(file path (use dialog)=w2388) -> (refnum out=w2387:refnum<file>, error out=w2386:errorcluster)  [unwired: 5 in, 1 out]
            n2055 = for {
              N: w2378 -> [_]
              tunnel: w2392 -> [w2507]
              tunnel: w2391 -> [w2506]
              tunnel: [w2496] -> w2358 mode=indexing
              tunnel: [w2494] -> w2356 mode=indexing
              tunnel: [w2495] -> w2351 mode=indexing
              tunnel: w2377 -> [_]
              tunnel: [w2488] -> w2353 mode=indexing
              tunnel: [w2484] -> w2329 mode=indexing
              tunnel: [w2480] -> w2304 mode=indexing
              tunnel: [w2476] -> w2285 mode=indexing
              tunnel: [w2471] -> w2243 mode=indexing
              (unwired) TRUE ("line mode (F)")
              n2056 = Read from Text File "Read File"(file (use dialog)=w2507, error in=w2506) -> (text=w2472:string)  [unwired: 2 in, 3 out]
              n2057 = local write "String 7"(w2472) -> ()
              n2058 = String Subset(string=w2472, offset (0)=85, length (rest)=9 ("length (rest)")) -> (substring=w2475:string)
              n2059 = String Subset(string=w2472, offset (0)=35, length (rest)=9 ("length (rest)")) -> (substring=w2497:string)
              n2060 = String Subset(string=w2472, offset (0)=55, length (rest)=9 ("length (rest)")) -> (substring=w2483:string)
              n2061 = String Subset(string=w2472, offset (0)=25, length (rest)=9 ("length (rest)")) -> (substring=w2477:string)
              n2062 = String Subset(string=w2472, offset (0)=45, length (rest)=9 ("length (rest)")) -> (substring=w2485:string)
              n2063 = String Subset(string=w2472, offset (0)=0, length (rest)=14 ("length (rest)")) -> (substring=w2500:string)
              n2064 = String Subset(string=w2472, offset (0)=15, length (rest)=9 ("length (rest)")) -> (substring=w2503:string)
              n2065 = String Subset(string=w2472, offset (0)=65, length (rest)=9 ("length (rest)")) -> (substring=w2489:string)
              n2066 = Fract/Exp String To Number(string=w2475) -> (number=w2471:dbl)  [unwired: 3 in, 1 out]
              n2067 = Fract/Exp String To Number(string=w2497) -> (number=w2495:dbl)  [unwired: 3 in, 1 out]
              n2068 = Fract/Exp String To Number(string=w2483) -> (number=w2480:dbl)  [unwired: 3 in, 1 out]
              n2069 = Fract/Exp String To Number(string=w2477) -> (number=w2476:dbl)  [unwired: 3 in, 1 out]
              n2070 = Fract/Exp String To Number(string=w2485) -> (number=w2484:dbl)  [unwired: 3 in, 1 out]
              n2071 = Fract/Exp String To Number(string=w2500) -> (number=w2496:dbl)  [unwired: 3 in, 1 out]
              n2072 = Fract/Exp String To Number(string=w2503) -> (number=w2494:dbl)  [unwired: 3 in, 1 out]
              n2073 = Fract/Exp String To Number(string=w2489) -> (number=w2492:dbl)  [unwired: 3 in, 1 out]
              n2074 = Add(x=w2492, y=0.0) -> (x+y=w2488:dbl)
            }
            n2075 = for {
              N: w2380 -> [_]
              tunnel: w2387 -> [w2435]
              tunnel: w2386 -> [w2434]
              tunnel: [w2424] -> w2340 mode=indexing
              tunnel: [w2423] -> w2333 mode=indexing
              tunnel: w2377 -> [_]
              tunnel: [w2412] -> w2338 mode=indexing
              tunnel: [w2417] -> w2335 mode=indexing
              tunnel: [w2413] -> w2325 mode=indexing
              tunnel: [w2408] -> w2300 mode=indexing
              tunnel: [w2404] -> w2281 mode=indexing
              tunnel: [w2399] -> w2241 mode=indexing
              (unwired) 1.0 ("x")
              (unwired) TRUE ("line mode (F)")
              n2076 = Read from Text File "Read File"(file (use dialog)=w2435, error in=w2434) -> (text=w2400:string)  [unwired: 2 in, 3 out]
              n2077 = local write "String 12"(w2400) -> ()
              n2078 = String Subset(string=w2400, offset (0)=85, length (rest)=9 ("length (rest)")) -> (substring=w2402:string)
              n2079 = String Subset(string=w2400, offset (0)=35, length (rest)=9 ("length (rest)")) -> (substring=w2425:string)
              n2080 = String Subset(string=w2400, offset (0)=55, length (rest)=9 ("length (rest)")) -> (substring=w2410:string)
              n2081 = String Subset(string=w2400, offset (0)=25, length (rest)=9 ("length (rest)")) -> (substring=w2406:string)
              n2082 = String Subset(string=w2400, offset (0)=45, length (rest)=9 ("length (rest)")) -> (substring=w2415:string)
              n2083 = String Subset(string=w2400, offset (0)=15, length (rest)=9 ("length (rest)")) -> (substring=w2431:string)
              n2084 = String Subset(string=w2400, offset (0)=0, length (rest)=14 ("length (rest)")) -> (substring=w2428:string)
              n2085 = String Subset(string=w2400, offset (0)=65, length (rest)=9 ("length (rest)")) -> (substring=w2418:string)
              n2086 = Fract/Exp String To Number(string=w2402) -> (number=w2399:dbl)  [unwired: 3 in, 1 out]
              n2087 = Fract/Exp String To Number(string=w2425) -> (number=w2423:dbl)  [unwired: 3 in, 1 out]
              n2088 = Fract/Exp String To Number(string=w2410) -> (number=w2408:dbl)  [unwired: 3 in, 1 out]
              n2089 = Fract/Exp String To Number(string=w2406) -> (number=w2404:dbl)  [unwired: 3 in, 1 out]
              n2090 = Fract/Exp String To Number(string=w2415) -> (number=w2413:dbl)  [unwired: 3 in, 1 out]
              n2091 = Fract/Exp String To Number(string=w2431) -> (number=w2412:dbl)  [unwired: 3 in, 1 out]
              n2092 = Fract/Exp String To Number(string=w2428) -> (number=w2424:dbl)  [unwired: 3 in, 1 out]
              n2093 = Fract/Exp String To Number(string=w2418) -> (number=w2421:dbl)  [unwired: 3 in, 1 out]
              n2094 = Add(x=w2421, y=0.0) -> (x+y=w2417:dbl)
            }
            n2095 = Delete From Array(array=w2283, index=0) -> (array with subset deleted=w2256:dbl[])  [unwired: 1 in, 1 out]
            n2096 = Delete From Array(array=w2346, index=0) -> (array with subset deleted=w2319:dbl[])  [unwired: 1 in, 1 out]
            n2097 = Delete From Array(array=w2326, index=0) -> (array with subset deleted=w2314:dbl[])  [unwired: 1 in, 1 out]
            n2098 = Delete From Array(array=w2344, index=0) -> (array with subset deleted=w2345:dbl[])  [unwired: 1 in, 1 out]
            n2099 = call-poly <vilib>:"Mean.vi"("X"=w2256) -> ("mean"=→"КОФ2 4":dbl)  [unwired: 1 out]
            n2100 = call-poly <vilib>:"Mean.vi"("X"=w2319) -> ("mean"=→"КОФ3":dbl)  [unwired: 1 out]
            n2101 = call-poly <vilib>:"Mean.vi"("X"=w2314) -> ("mean"=→"CP3":dbl)  [unwired: 1 out]
            n2102 = Delete From Array(array=w2308, index=0) -> (array with subset deleted=w2235:dbl[])  [unwired: 1 in, 1 out]
            n2103 = Delete From Array(array=w2247, index=0) -> (array with subset deleted=w2234:dbl[])  [unwired: 1 in, 1 out]
            n2104 = Delete From Array(array=w2287, index=0) -> (array with subset deleted=w2258:dbl[])  [unwired: 1 in, 1 out]
            n2105 = Delete From Array(array=w2365, index=0) -> (array with subset deleted=w2320:dbl[])  [unwired: 1 in, 1 out]
            n2106 = Delete From Array(array=w2331, index=0) -> (array with subset deleted=w2316:dbl[])  [unwired: 1 in, 1 out]
            "array w/ subset deleted" <- w2316
            n2107 = Delete From Array(array=w2362, index=0) -> (array with subset deleted=w2363:dbl[])  [unwired: 1 in, 1 out]
            n2108 = call-poly <vilib>:"Mean.vi"("X"=w2258) -> ("mean"=→"КОФ2 2":dbl)  [unwired: 1 out]
            n2109 = call-poly <vilib>:"Mean.vi"("X"=w2320) -> ("mean"=→"КОФ1":dbl)  [unwired: 1 out]
            n2110 = Bundle "Bundle"(w2235, w2234) -> (w2240:cluster{dbl[], dbl[]})  [unwired: 1 in]
            n2111 = Bundle "Bundle"(w2235, w2363) -> (w2227:cluster{dbl[], dbl[]})  [unwired: 1 in]
            n2112 = Delete From Array(array=w2242, index=0) -> (array with subset deleted=w2230:dbl[])  [unwired: 1 in, 1 out]
            n2113 = Delete From Array(array=w2243, index=0) -> (array with subset deleted=w2232:dbl[])  [unwired: 1 in, 1 out]
            n2114 = Delete From Array(array=w2353, index=0) -> (array with subset deleted=w2354:dbl[])  [unwired: 1 in, 1 out]
            n2115 = Delete From Array(array=w2241, index=0) -> (array with subset deleted=w2228:dbl[])  [unwired: 1 in, 1 out]
            n2116 = Delete From Array(array=w2335, index=0) -> (array with subset deleted=w2336:dbl[])  [unwired: 1 in, 1 out]
            n2117 = Delete From Array(array=w2360, index=0) -> (array with subset deleted=w2266:dbl[])  [unwired: 1 in, 1 out]
            n2118 = Delete From Array(array=w2306, index=0) -> (array with subset deleted=w2262:dbl[])  [unwired: 1 in, 1 out]
